vi "list and create PG alarms sequence_1.vi"(8 "error in":errorcluster, 9 "sequence name trunc":string, 10 "sequence name curr":string, 11 "conn":u32) -> (0 "error out":errorcluster, 3 "conn_out":u32)   [LabVIEW 2019, in "PostgreSQL.lvlib"]
uses:
  PostgreSQL.lvlib
  PostgreSQL2LabVIEW/libpqlv/src/PQresultErrorMessage.vi
  PostgreSQL2LabVIEW/libpqUtility/src/PQclear.vi
  PostgreSQL2LabVIEW/libpqlv/src/PQsendQuery.vi
  PostgreSQL2LabVIEW/libpqlv/src/PQgetResult.vi
  PostgreSQL2LabVIEW/libpqlv/src/PQresultStatus.vi
  PostgreSQL2LabVIEW/libpqUtility/src/PQgetColumn.vi
  PostgreSQL2LabVIEW/libpqlv/src/PQclear.vi
  PostgreSQL2LabVIEW/libpqUtility/src/PQfetchTables.vi
  PostgreSQL2LabVIEW/libpqlv/src/PQgetvalue.vi
  PostgreSQL2LabVIEW/libpqlv/src/PQntuples.vi
  PostgreSQL2LabVIEW/libpqUtility/libpqutility.lvlib
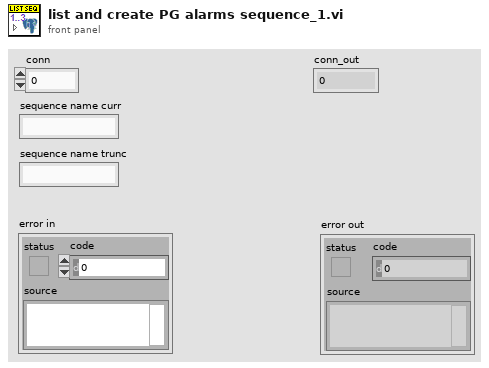
[diagram p1: front panel]
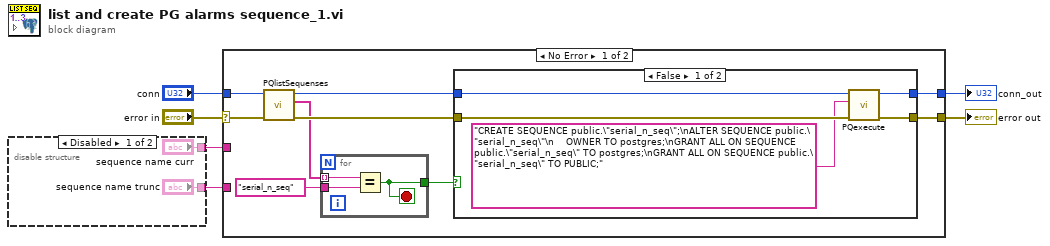
[diagram p0: block diagram]
diagram:
  n1 = disable-structure shown="Disabled" {
    disable-tunnel: ["sequence name curr" _] -> w2
    disable-tunnel: ["sequence name trunc" _] -> w1
    frame Disabled {
    }
    frame Enabled {
    }
  }
  n2 = case shown="No Error" "error in" {
    selector: "error in" -> [w14 w29]
    tunnel: "conn" -> [w11 w28]
    tunnel: [w17 w28] -> w4
    tunnel: [w16 w29] -> w3
    tunnel: w2 -> [_ _]
    tunnel: w1 -> [_ _]
    frame No Error {
      n3 = call "PQlistSequenses.vi"("error in"=w14, "conn"=w11) -> ("error out"=w13:errorcluster, "Data"=w10:string[], "conn_out"=w12:u32)  [unwired: 7 in]
      n4 = for {
        tunnel: "serial_n_seq" -> [w19]
        tunnel: w10 -> [w20] mode=indexing
        tunnel: [w18] -> w15
        stop <- w18 stop-if-true
        n5 = Equal?(x=w20, y=w19) -> (x = y?=w18:bool)
      }
      n6 = case shown="False" w15 {
        tunnel: w12 -> [w25 w27]
        tunnel: [w23 w27] -> w17
        tunnel: w13 -> [w24 w26]
        tunnel: [w22 w26] -> w16
        frame False {
          n7 = call "PQexecute.vi"("error in"=w24, "SQL querry"="CREATE SEQUENCE public.\"serial_n_seq\";\nALTER SEQUENCE public.\"serial_n_seq\"\n    OWNER TO postgres;\nGRANT ALL ON SEQUENCE public.\"serial_n_seq\" TO postgres;\nGRANT ALL ON SEQUENCE public.\"serial_n_seq\" TO PUBLIC;", "conn"=w25) -> ("error out"=w22:errorcluster, "conn_out"=w23:u32)  [unwired: 7 in]
        }
        frame True {
        }
      }
    }
    frame Error {
    }
  }
  "conn_out" <- w4
  "error out" <- w3
